vi "Randomizer.vi"(8 "error in":errorcluster, 10 "Difficulty":i32, 11 "Commands":T2=enum."Initialize") -> (0 "error out":errorcluster, 3 "Facets To move":T1[](array[typedef]))   [LabVIEW 2019]
uses:
  Play timing module commands.ctl
  Rubix Array data type.ctl
  <vilib>/Platform/TimedLoop/XDataNode/timing_clust.ctl
  <vilib>/Platform/TimedLoop/XDataNode/nitl_modes.ctl
  <vilib>/Platform/TimedLoop/XDataNode/wakeup.ctl
  Cube Data Ops.ctl
  <vilib>/Platform/TimedLoop/scheduler/LVUserAPI/_suppVIs/Create_1kHz_TSource.vi
  preform rotate op -numeric.vi
  <vilib>/Platform/TimedLoop/XDataNode/XDataNode.xnode
  <vilib>/Platform/TimedLoop/XDataNode/XDNodeRunTimeDep.lvlib
panel:
  # "Ajout Juliette"
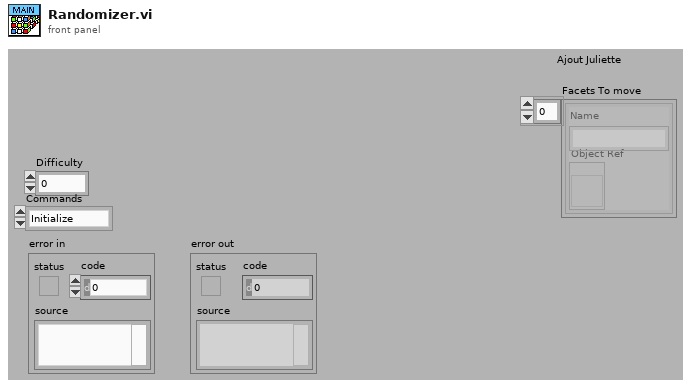
[diagram p1: front panel]
types:
  T1 = typedef "Rubix Array data type.ctl" = cluster{"Object Ref":refnum<vi>, "Name":string}
  T2 = typedef "Play timing module commands.ctl" = enum16{"Clean up", "Initialize", "Run"}
  T3 = typedef "Cube Data Ops.ctl" = enum16{"Initialize", "Set Rubix Ref Array", "Set Rubix Text Array", "Set Current Face", "Get Rubix Text Array", "Generate Rubix Array", "Get Rubix array", "Get Facets to move", "Randomize", "Top row left", "Top row right", "Middle row left", "Middle row right", "Bottom row left", "Bottom row right", "Left column up", "Left column down", "Middle column up", "Middle column down", "Right column up", "Right column down", "Face ccw", "Face cw"}
  T4 = typedef "XDNodeRunTimeDep.lvlib/timing_clust.ctl" = cluster{"Expected End [f-1]":u64, "Actual End [f-1]":u64, "Finished Late? [f-1]":bool, "Expected End [i-1]":u64, "Actual End [i-1]":u64, "Finished Late? [i-1]":bool, "Expected Start [i]":u64, "Actual Start [i]":u64, "Expected Start [f]":u64, "Actual Start [f]":u64, "Source Name":string, "Structure Name":string, "Period":i64, "Deadline":i64, "Offset":i64, "Start":i64, "Priority":i32, "Timeout":i32, "Mode":T5, "Wakeup Reason":T6, "Error":errorcluster, "Source Type":string, "Secondary Source Type":string, "Global End Time":u64, "Global Start Time":u64, "Frame Duration":u64, "Iteration Duration":u64, "Assigned CPU":i32, "I/O Scan Engine Mode":u32}
  T5 = typedef "XDNodeRunTimeDep.lvlib/nitl_modes.ctl" = enum32{"No Change", "Process missed periods, maintain original phase", "Discard missed periods, maintain original phase", "Process missed periods, ignore original phase", "Discard missed periods, ignore original phase"}
  T6 = typedef "XDNodeRunTimeDep.lvlib/wakeup.ctl" = enum32{"Normal", "Aborted", "Asynchronous wakeup", "Timing source error", "Timed loop error", "Timeout"}
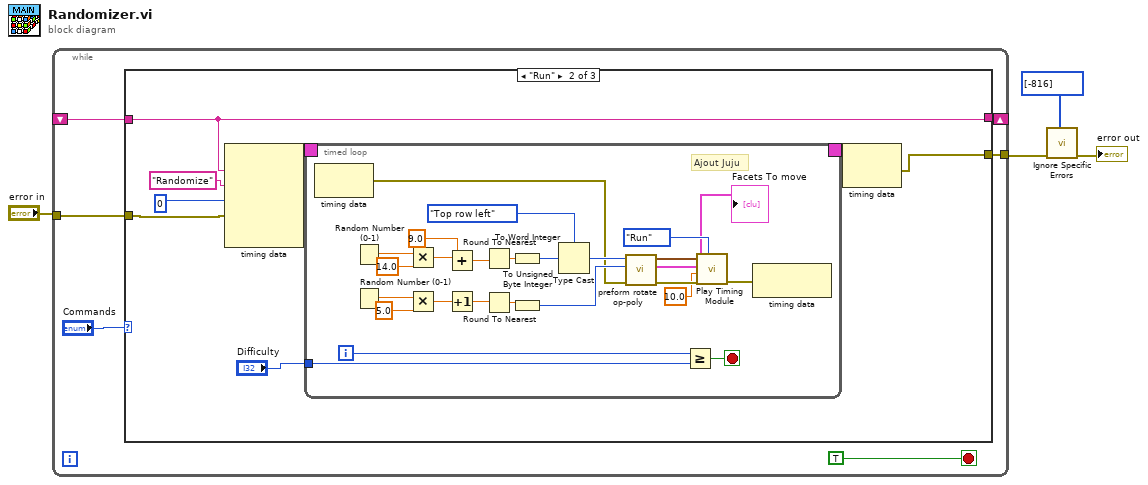
[diagram p0: block diagram]
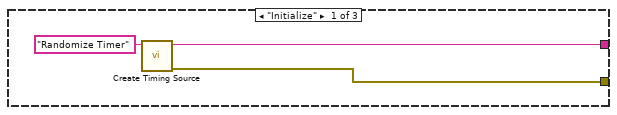
[diagram p2: hidden frame]
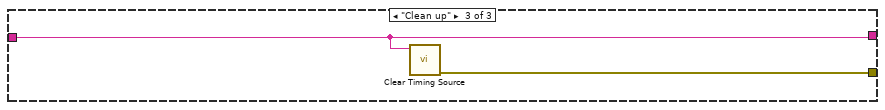
[diagram p3: hidden frame]
diagram:
  n1 = while {
    tunnel: [w9] -> w1
    shift-right: [w7] -> _
    shift-left: _ -> [w6]
    tunnel: "error in" -> [w5]
    stop <- TRUE stop-if-true
    n2 = case shown="\"Run\"" "Commands" {
      tunnel: [w11 w17 w60] -> w9
      tunnel: [w13 w15 w61] -> w7
      tunnel: w6 -> [_ w15 w61]
      tunnel: w5 -> [_ w14 _]
      frame "Initialize" {
        n3 = call-poly <vilib>:"Create Timing Source.vi"("name (in)"="Randomize Timer") -> ("error out"=w11:errorcluster, "name (out)"=w13:string)  [unwired: 9 in]
      }
      frame "Run" {
        n4 = node-c288(w15, "Randomize" ("Name"), i64 0 ("Period"), w14) -> (w21:T4)  [unwired: 1 in]
        n5 = timed-loop {
          timing: w21 -> [_]
          timing-out: [_] -> w20
          tunnel: "Difficulty" -> [w27]
          i -> [w25]
          stop <- w26 stop-if-true
          # "Ajout Juju"
          n6 = node-c288() -> (w23:errorcluster)  [unwired: 1 in]
          n7 = Random Number (0-1)() -> (number: 0 to 1=w42:dbl)
          n8 = Random Number (0-1)() -> (number: 0 to 1=w46:dbl)
          n9 = Multiply(x=w42, y=14.0) -> (x*y=w40:dbl)
          n10 = Multiply(x=w46, y=5.0) -> (x*y=w44:dbl)
          n11 = Add(x=w40, y=9.0) -> (x+y=w38:dbl)
          n12 = Increment(x=w44) -> (x+1=w43:dbl)
          n13 = Round To Nearest(number=w38) -> (nearest integer value=w35:dbl)
          n14 = Round To Nearest(number=w43) -> (nearest integer value=w34:dbl)
          n15 = To Word Integer(number=w35) -> (16bit integer=w37:i16)
          n16 = To Unsigned Byte Integer(number=w34) -> (unsigned 8bit integer=w33:u8)
          n17 = Type Cast(type=Cube_Data_Ops."Top row left" ("Rotate command"), x=w37) -> (*(type *) &x=w32:T3)
          n18 = call-poly "preform rotate op-poly.vi"("error in (no error)"=w23, "Face to act on"=w33, "Rotate command"=w32) -> ("error out(no error)"=w29:errorcluster, "Facets To move"=w22:T1[], "Axis"=w30:cluster{"X":sgl, "Y":sgl, "Z":sgl})  [unwired: 6 in]
          "Facets To move" <- w22
          n19 = Greater Or Equal?(x=w25, y=w27) -> (x >= y?=w26:bool)
          n20 = call "Play Timing Module.vi"("Commands"=Play_timing_module_commands."Run", "error in"=w29, "Rotation Resolution"=10.0, "Facets To move"=w22, "Axis"=w30) -> ("error out"=w24:errorcluster)  [unwired: 6 in]
          n21 = node-c288(w24) -> ()  [unwired: 1 out]
        }
        n22 = node-c288(w20) -> (w17:errorcluster)
      }
      frame "Clean up" {
        n23 = call <vilib>:"Clear Timing Source.vi"("name"=w61) -> ("error out"=w60:errorcluster)  [unwired: 9 in, 1 out]
      }
    }
  }
  n24 = call "Ignore Specific Errors.vi"("error in (no error)"=w1, "Array"=i32[] [-816]) -> ("error out"=→"error out":errorcluster)  [unwired: 8 in, 1 out]
